vi "StateSpaceModel.vi"(6 "dbp":dbl=0.05 caption="Пульсации в полосе\nподавления dbp [db]", 7 "dbs":dbl=120.0 caption="Пульсации в полосе\nпропускания dbs, [db]", 8 "f_cut":dbl=10.0 caption="Частота среза f_cut [Hz]", 9 "n":i32=3 caption="Порядок фильтра n") -> (0 "D":dbl[][](array[numeric]), 1 "C":dbl[][](array[numeric]), 2 "B":dbl[][](array[numeric]), 3 "A":dbl[][](array[numeric]), 4 "State-Space Model":T1 {"Transport Delay" format="%.2f"; "D" format="%#.2g"; "C" format="%#.2g"; "B" format="%#.2g"; "A" format="%#.2g"; "properties"."Sampling Time" format="%#.6p"; "properties"."Output Delays" format="%.4f"; "properties"."Input Delays" format="%.4f"})   [LabVIEW 2019]
uses:
  <vilib>/addons/Control Design/_Model Construction/Model Typedefs.llb/CD State Space Model (MIMO).ctl
  <vilib>/addons/Control Design/_Model Construction/Model Typedefs.llb/CD General Elements.ctl
  <vilib>/imath/engines/lvmath2/RunTimeEngine/BuiltInFunctions/iir_elliptic/NIMS_[4o]_iir_elliptic(I32,DBL2,V,Str).vi
  <vilib>/imath/engines/lvmath2/RunTimeEngine/ErrorHandling/NIMS_Create Error From Enums.vi
  <vilib>/imath/engines/lvmath/Plug In/Control Design/BuiltInFunctions/ss/NIMS_CD_ss(A,B,C,D).vi
  <vilib>/imath/engines/lvmath2/RunTimeEngine/NodeEndStatement/NIMS_NodeEndStatement_Output.vi
  <instcachedir>/0/NIMS_NodeEndStatement_Output_53EC0D466D134D7ABD903AC30B43404B.lvgen/NIMS_NodeEndStatement_Output_53EC0D466D134D7ABD903AC30B43404B_002.vi
  <instcachedir>/0/NIMS_NodeEndStatement_Output_53EC0D466D134D7ABD903AC30B43404B.lvgen/NIMS_NodeEndStatement_Output_53EC0D466D134D7ABD903AC30B43404B_011.vi
  <vilib>/imath/engines/lvmath2/RunTimeEngine/ErrorHandling/NIMS_Finalize Error.vi
  <vilib>/addons/Control Design/_Model Construction/NI_LinSys_Model Typedefs.lvlib
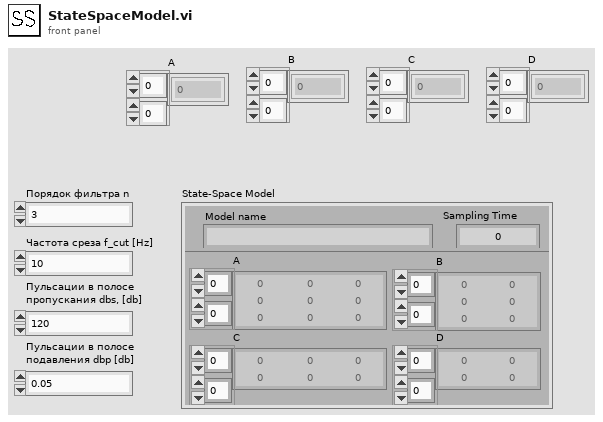
[diagram p1: front panel]
types:
  T1 = typedef "NI_LinSys_Model Typedefs.lvlib/CD State Space Model (MIMO).ctl" = cluster{"properties":T2, "A":dbl[][], "B":dbl[][], "C":dbl[][], "D":dbl[][], "StateNames":string[], "Transport Delay":dbl[][]}
  T2 = typedef "NI_LinSys_Model Typedefs.lvlib/CD General Elements.ctl" = cluster{"Model name":string, "Input names":string[], "Output names":string[], "Input Delays":dbl[], "Output Delays":dbl[], "Sampling Time":dbl, "Notes":string}
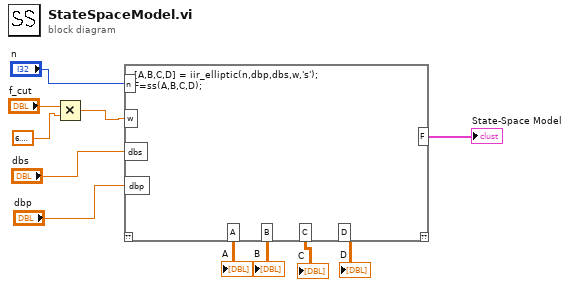
[diagram p0: block diagram]
diagram:
  n1 = Multiply(x="f_cut", y=6.283185307179586) -> (x*y=w8:dbl)
  n2 = mathscript code="[A,B,C,D] = iir_elliptic(n,dbp,dbs,w,'s');\nF=ss(A,B,C,D);"("n"="n", "w"=w8, "dbs"="dbs", "dbp"="dbp") -> ("F"=→"State-Space Model":T1, "A"=→"A":dbl[][], "B"=→"B":dbl[][], "C"=→"C":dbl[][], "D"=→"D":dbl[][])  [unwired: 1 in, 1 out]
